vi "Vision Research Phantom Series PhCon PhNVMGetStatus.vi"(0 "CN in":u32=1, 1 "pCineCnt":u32, 5 "Error In (no error)":errorcluster) -> (14 "CN out":u32=1, 15 "pCineCnt out":u32, 17 "pTime":i32[](array[numeric]), 18 "pFreeSp":u32, 19 "Error Out":errorcluster)   [LabVIEW 2013, in "VRI.lvlib"]
doc: "PhCon.dll\n\nPhNVMGetStatus\nHRESULT PhNVMGetStatus (UINT CN, PUINT pCineCnt, time_t *pTime, PUINT pFreeSp);\n\nParameters Description\nCN (in) Camera number.\npCineCnt (in,out) At input: the size of the array, at output the count of cines stored in NV memory\npTime (out) Array with the trigger time for each cine\npFreeSp (out) Free space in NVM in MB\nReturn HRESULT (0=Ok)\nComments Get the trigger time of the specified cine stored in the nonvolatile memory.\n It can be used in the user interface to allow the user to select the cine to be \n restored from NonVolatile memory\n\nWritten by:\nBLOOMY CONTROLS, INC\nWINDSOR, CT 06095, USA\n860-298-9925\nwww.bloomy.com\nV1.0.0\nMay, 2004"
uses:
  VRI.lvlib
  Phantom DLLs/PhCon.dll
panel:
  # "For instructions on the use of this VI, press Ctrl+H to display the help window and move the mouse over the icon, controls, and indicators"
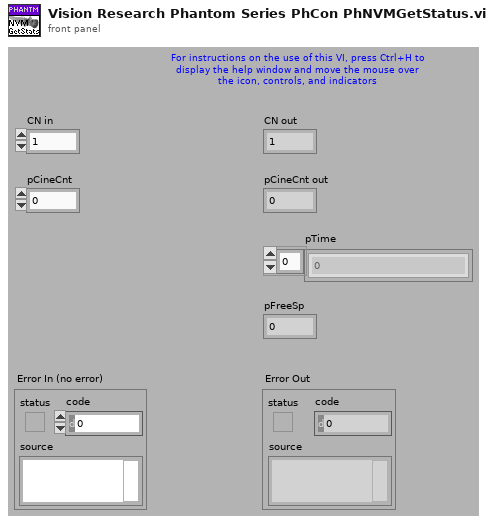
[diagram p1: front panel]
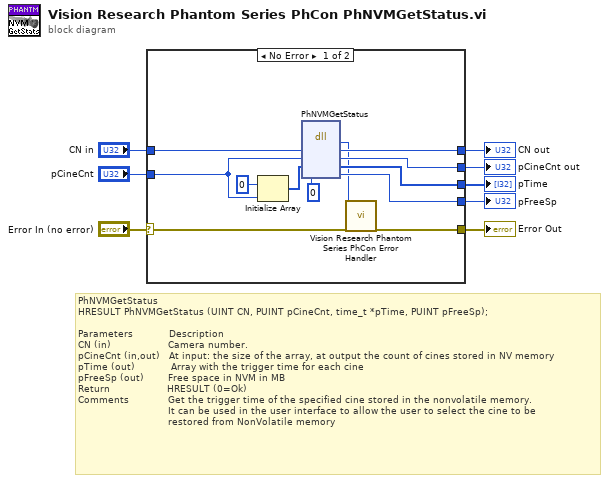
[diagram p0: block diagram]
diagram:
  # "PhNVMGetStatus\nHRESULT PhNVMGetStatus (UINT CN, PUINT pCineCnt, time_t *pTime, PUINT pFreeSp);\n\nParameters            Description\nCN (in)                   Camera number.\npCineCnt (in,out)   At input: the size of the array, at output the count of cines stored in NV memory\npTime (out)            Array with the trigger time for each cine\npFreeSp (out)        Free space in NVM in MB\nReturn                   HRESULT (0=Ok)\nComments             Get the trigger time of the specified cine stored in the nonvolatile memory.\n                              It can be used in the user interface to allow the user to select the cine to be \n                              restored from NonVolatile memory"
  n1 = case shown="No Error" "Error In (no error)" {
    selector: "Error In (no error)" -> [w20 w22]
    tunnel: [w19 w22] -> w7
    tunnel: "CN in" -> [w18 w21]
    tunnel: [w17 w21] -> w5
    tunnel: "pCineCnt" -> [w16 _]
    tunnel: [w15 _] -> w3
    tunnel: [w14 _] -> w2
    tunnel: [w13 _] -> w1
    frame No Error {
      n2 = Initialize Array(u32 0 ("element"), w16) -> (w11:u32[])
      n3 = dll-call lib="C:/Projects/SDK/32-bit/Vision Research Phantom Series Labview Driver/Phantom DLLs/PhCon.dll" fn="PhNVMGetStatus"("CN"=w18, "pCineCnt"=w16, "pTime"=w11, "pFreeSp"=u32 0) -> ("HRESULT"=w12:i32, "CN"=w17:u32, "pCineCnt"=w15:u32, "pTime"=w14:u32[], "pFreeSp"=w13:u32)  [unwired: 3 in, 2 out]
      n4 = call "Vision Research Phantom Series PhCon Error Handler.vi"("ErrNo"=w12, "Error In (no error)"=w20) -> ("Error Out"=w19:errorcluster)  [unwired: 17 out]
    }
    frame Error {
    }
  }
  "Error Out" <- w7
  "CN out" <- w5
  "pTime" <- w2
  "pCineCnt out" <- w3
  "pFreeSp" <- w1
